vi "Dll Path.vi"() -> (3 "Dll path":path)   [LabVIEW 2019, in "Lab Streaming Layer.lvlib"]
uses:
  Lab Streaming Layer.lvlib
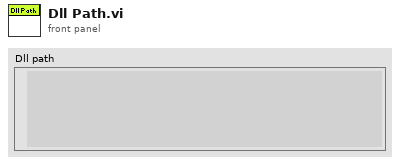
[diagram p1: front panel]
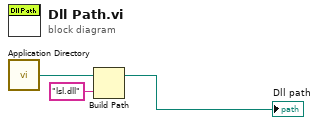
[diagram p0: block diagram]
diagram:
  n1 = call <vilib>:"Application Directory.vi"() -> ("Application Directory"=w3:path)
  n2 = Build Path(base path=w3, name or relative path="lsl.dll") -> (appended path=→"Dll path":path)
